vi "Efield_compute_2024lv.vi"() -> ()   [LabVIEW 2024]
panel:
  out "Efield":dbl
  in  "d_top":dbl format="%#_13g"
  in  "d_bottom":dbl format="%#_13g"
  in  "V_top":dbl format="%#_13g"
  in  "V_bottom":dbl format="%#_13g"
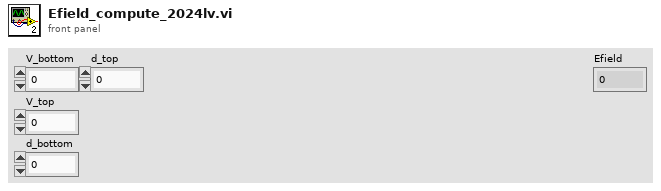
[diagram p1: front panel]
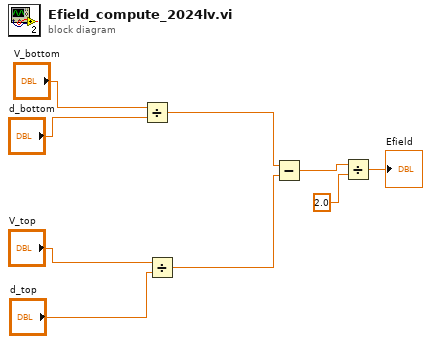
[diagram p0: block diagram]
diagram:
  n1 = Divide(x="V_bottom", y="d_bottom") -> (x/y=w5:dbl)
  n2 = Divide(x="V_top", y="d_top") -> (x/y=w4:dbl)
  n3 = Subtract(x=w5, y=w4) -> (x-y=w3:dbl)
  n4 = Divide(x=w3, y=2.0) -> (x/y=→"Efield":dbl)
